vi "4_Meas_Tdon.vi"(5 "Request #":string, 6 "TEST #":string, 7 "Project #":string, 8 "error in (no error)":errorcluster, 9 "ICE":dbl, 10 "VGE":dbl, 11 "file path (IN)":path) -> (0 "error out":errorcluster, 1 "DONE Tdon":bool, 2 "Tdon (ns)":dbl, 3 "file path (OUT)":path, 4 "ON Region":waveform(dbl)[](graph) caption="Tdon (ns)")   [LabVIEW 2020]
uses:
  <vilib>/Waveform/WDTOps.llb/WDT Waveform Duration DBL.vi
  <vilib>/Waveform/WDTOps.llb/WDT Get Waveform Subset DBL.vi
  <vilib>/measure/mascope.llb/Transition Measurements 1 chan.vi
  <vilib>/measure/NI_MAPro.lvlib
panel:
  out "Cursor a : Channel 2":dbl
  out "Cursor a : Channel 1":dbl
  in  "Decision ?":bool
  in  "Cursor a : Channel 1 \nrise edge tolerance":dbl=0.1
  in  "Cursor a : Channel 1 \nrise edge number":i32=1
  in  "Cursor a : Channel 2\nrise edge tolerance":dbl=0.1
  in  "Cursor a : Channel 2\nrise edge number":i32=1
  in  "reference  levels (CH1 initialize)":T1={"high ref level"=90.0, "mid ref level"=50.0, "low ref level"=10.0, "ref units"=1} {"ref units" items=["absolute", "percent"]; "high ref level" format="%0.2f"; "low ref level" format="%0.2f"; "mid ref level" format="%0.2f"}
  in  "reference  levels (CH2 initialize)":T1={"high ref level"=90.0, "mid ref level"=50.0, "low ref level"=10.0, "ref units"=1} {"ref units" items=["absolute", "percent"]; "high ref level" format="%0.2f"; "low ref level" format="%0.2f"; "mid ref level" format="%0.2f"}
  out "measurement info (CH2)":T2 {"ref levels"."ref units" items=["absolute", "relative"]; "ref levels"."high ref level" format="%.2p"; "ref levels"."low ref level" format="%.2p"; "ref levels"."mid ref level" format="%.2p"; "end time" format="%.6e"; "start time" format="%.6e"}
  out "measurement info (CH1)":T2 {"ref levels"."ref units" items=["absolute", "relative"]; "ref levels"."high ref level" format="%.2p"; "ref levels"."low ref level" format="%.2p"; "ref levels"."mid ref level" format="%.2p"; "end time" format="%.6e"; "start time" format="%.6e"}
  out "10% Vge":dbl
  out "10% Ice":dbl
  out "Waveform Graph":waveform(dbl)[](graph)
  # "From 10% Vge to 10% Ice"
  # "\"ON Region\" Test"
  # "From 10% Vge to 10% Ice"
  # "Default = 1"
  # "Default = 1"
  # "Default = 0.1"
  # "Default = 0.1"
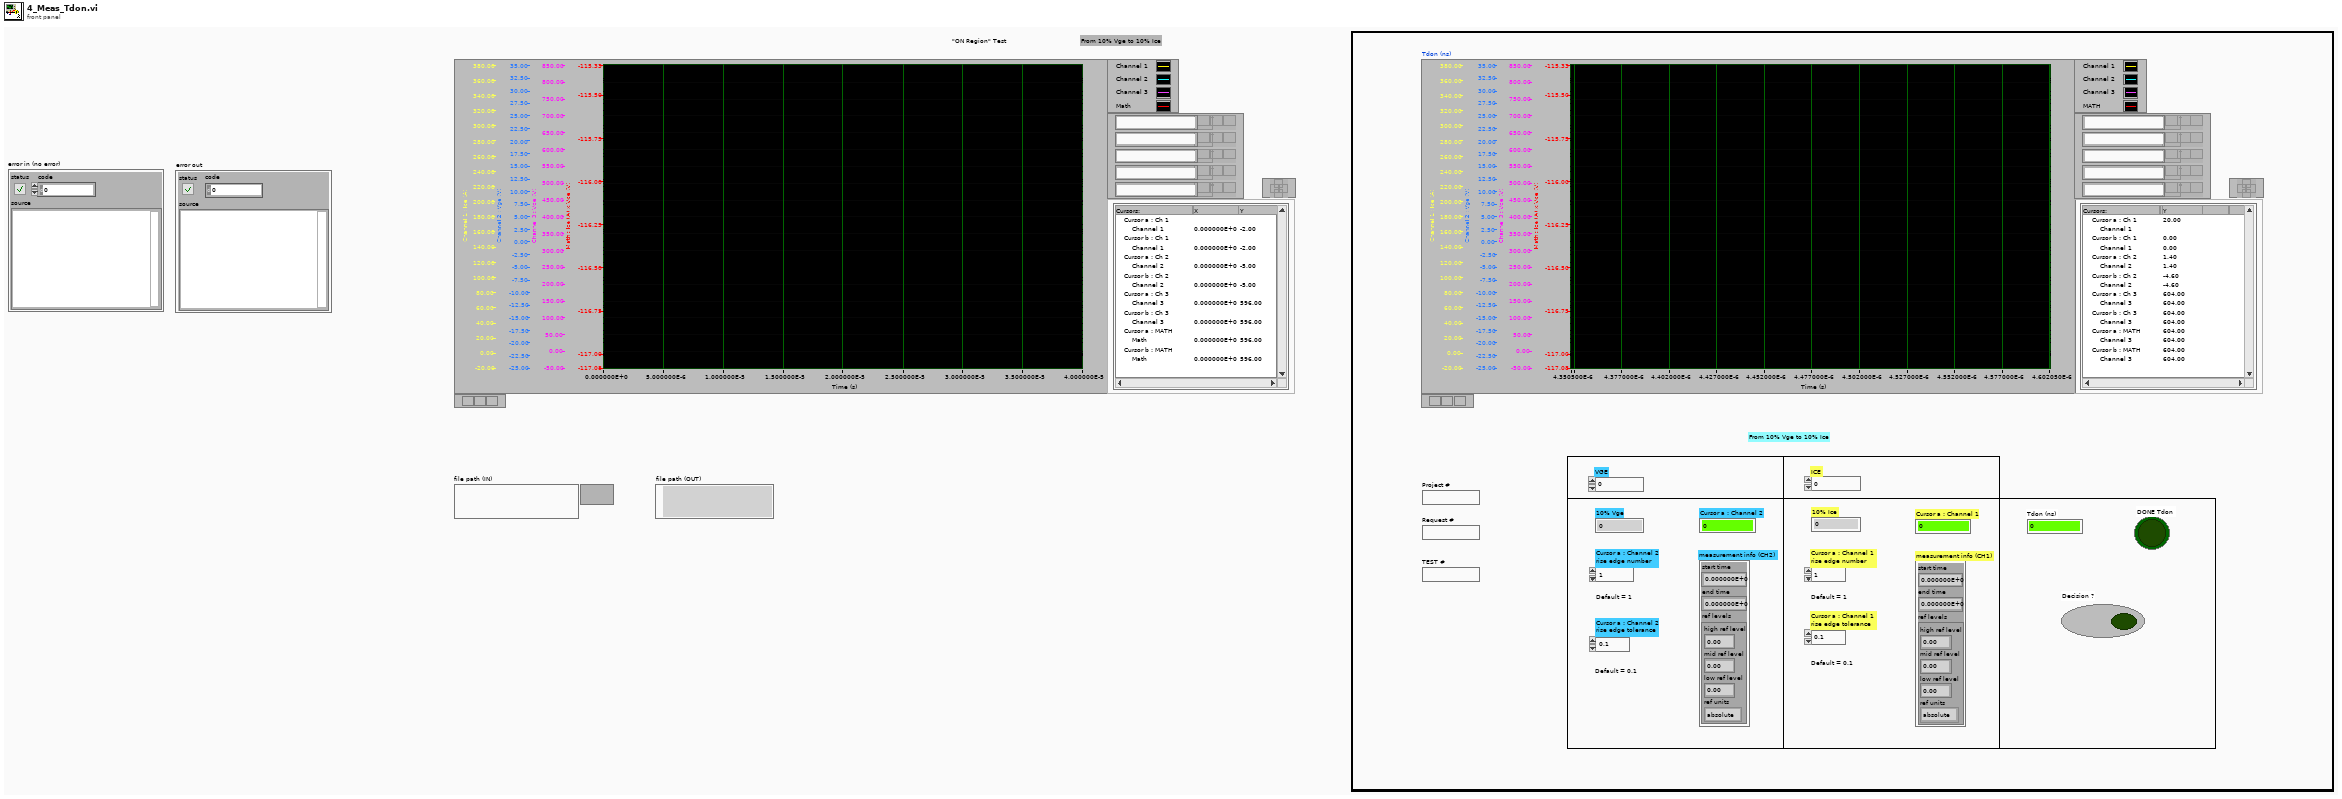
[diagram p1: front panel]
types:
  T1 = cluster{"high ref level":dbl, "mid ref level":dbl, "low ref level":dbl, "ref units":u16}
  T2 = cluster{"start time":dbl, "end time":dbl, "ref levels":cluster{"high ref level":dbl, "mid ref level":dbl, "low ref level":dbl, "ref units":u16}}
  T3 = enum32{"Invalid", "Standard", "Closed", "Hidden", "Minimized", "Maximized"}
  T4 = typedef "imagedata.ctl" = cluster{"image type":i32, "image depth":i32, "image":u8[], "mask":u8[], "colors":u32[], "Rectangle":cluster{"left":i16, "top":i16, "right":i16, "bottom":i16}}
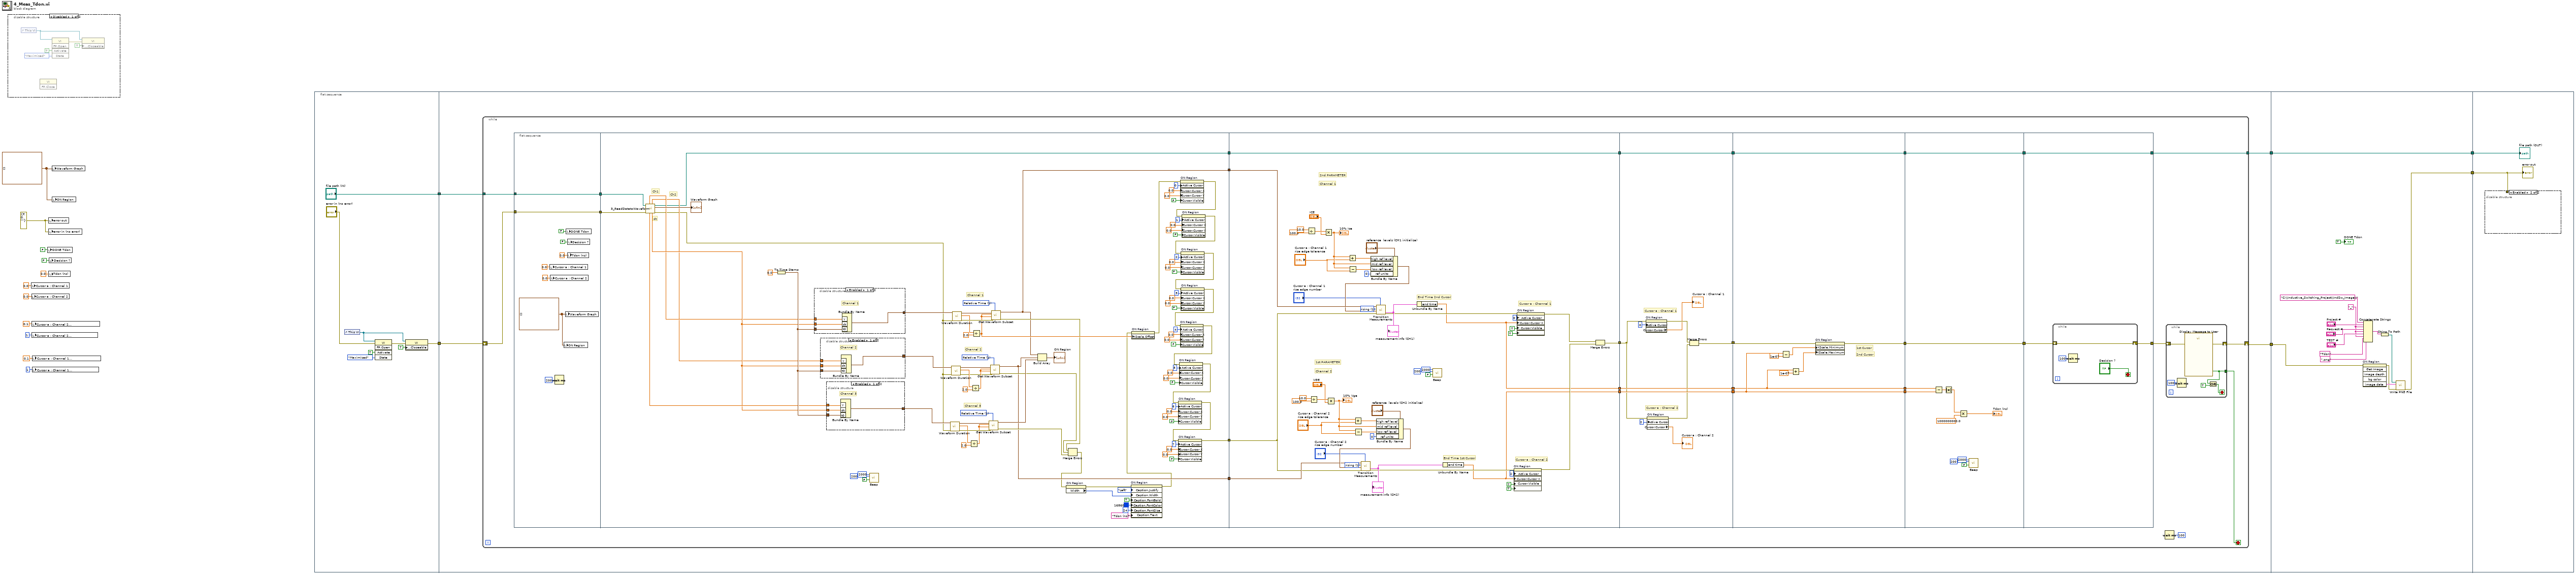
[diagram p0: block diagram]
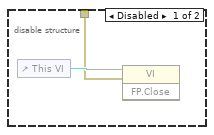
[diagram p6: hidden frame]
diagram:
  w16 = errorcluster {"status"=FALSE, "code"=0, "source"=""} ("error out")
  w17 = waveform(dbl)[] [] ("Waveform Graph")
  n1 = disable-structure shown="Disabled" {
    frame Disabled {
      n2 = control-ref of="This VI"() -> (w19:refnum<vi>)
      n3 = invoke class="VI" method="FP.Close"() -> (reference=w18:refnum<vi>)  [unwired: 2 in, 3 out]
      n4 = invoke class="VI" method="FP.Open"(reference=w19, "Activate"=TRUE ("Activate?"), "State"=T3."Maximized") -> (error in=w22:errorcluster, error out=w20:errorcluster)  [unwired: 1 in, 4 out]
      n5 = property class="VI"(reference=w19, error in=w20, "Front Panel.Closeable"=TRUE ("Front Panel Window:Closeable")) -> ()  [unwired: 2 out]
    }
    frame Enabled {
    }
  }
  n6 = local write "Cursor a : Channel 1"(0.0 ("Cursor a : Channel 1")) -> ()
  n7 = local write "Cursor a : Channel 2"(0.0 ("Cursor a : Channel 2")) -> ()
  n8 = local write "Cursor a : Channel 2\nrise edge tolerance"(0.1 ("Cursor a : Channel 2\nrise edge tolerance")) -> ()
  n9 = local write "Cursor a : Channel 2\nrise edge number"(1 ("Cursor a : Channel 2\nrise edge number")) -> ()
  n10 = local write "Cursor a : Channel 1 \nrise edge tolerance"(0.1 ("Cursor a : Channel 1 \nrise edge tolerance")) -> ()
  n11 = local write "Cursor a : Channel 1 \nrise edge number"(1 ("Cursor a : Channel 1 \nrise edge number")) -> ()
  n12 = local write "DONE Tdon"(FALSE ("DONE Tdon")) -> ()
  n13 = local write "error out"(w16) -> ()
  n14 = local write "error in (no error)"(w16) -> ()
  n15 = local write "Tdon (ns)"(0.0 ("Tdon (ns)")) -> ()
  n16 = local write "Decision ?"(FALSE ("Decision ?")) -> ()
  n17 = local write "Waveform Graph"(w17) -> ()
  n18 = local write "ON Region"(w17) -> ()
  n19 = flat-sequence {
    tunnel: ["file path (IN)"] -> w6
    tunnel: [w27] -> w5
    tunnel: [w35] -> w15
    tunnel: [w34] -> w12
    tunnel: w6 -> [w36]
    tunnel: w5 -> [w33]
    tunnel: w15 -> [w270]
    tunnel: [w269] -> w14
    tunnel: [w268] -> w13
    tunnel: w12 -> [w268]
    tunnel: w14 -> [w283]
    tunnel: w13 -> [w284]
    frame #0 {
      n20 = control-ref of="This VI"() -> (w31:refnum<vi>)
      n21 = invoke class="VI" method="FP.Open"(reference=w31, error in="error in (no error)", "Activate"=TRUE ("Activate?"), "State"=T3."Maximized") -> (error out=w32:errorcluster)  [unwired: 1 in, 4 out]
      n22 = property class="VI"(reference=w31, error in=w32, "Front Panel.Closeable"=TRUE ("Front Panel Window:Closeable")) -> (error out=w27:errorcluster)  [unwired: 1 out]
    }
    frame #1 {
      n23 = while {
        tunnel: w36 -> [w52]
        shift-right: [w38] -> w35
        shift-left: w33 -> [w50]
        tunnel: [w48] -> w34
        stop <- w37 stop-if-true
        n24 = flat-sequence {
          tunnel: [w77] -> w63
          tunnel: [w78] -> w62
          tunnel: w52 -> [w78]
          tunnel: w50 -> [w77]
          tunnel: w63 -> [w170]
          tunnel: w62 -> [w164]
          tunnel: [w91] -> w61
          tunnel: [w90] -> w60
          tunnel: [w89] -> w59
          tunnel: [w79] -> w58
          tunnel: w61 -> [w207]
          tunnel: w60 -> [w206]
          tunnel: w59 -> [w205]
          tunnel: [w193] -> w47
          tunnel: [w192] -> w45
          tunnel: [w191] -> w43
          tunnel: w58 -> [w190]
          tunnel: [w190] -> w41
          tunnel: w47 -> [w241]
          tunnel: [w241] -> w46
          tunnel: w45 -> [w240]
          tunnel: [w240] -> w44
          tunnel: w43 -> [w235]
          tunnel: [w238] -> w42
          tunnel: w41 -> [w239]
          tunnel: [w239] -> w40
          tunnel: w46 -> [w242]
          tunnel: [w242] -> w57
          tunnel: w44 -> [w243]
          tunnel: [w243] -> w56
          tunnel: w42 -> [w249]
          tunnel: [w248] -> w55
          tunnel: w40 -> [w250]
          tunnel: [w250] -> w54
          tunnel: w57 -> [w260]
          tunnel: w56 -> [w259]
          tunnel: w55 -> [w252]
          tunnel: w54 -> [w251]
          tunnel: [w252] -> w53
          tunnel: [w251] -> w49
          tunnel: w53 -> [w264]
          tunnel: [w263] -> w39
          tunnel: w49 -> [w262]
          tunnel: [w262] -> w48
          frame #0 {
            w73 = waveform(dbl)[] [] ("Waveform Graph")
            n25 = local write "Cursor a : Channel 1"(0.0 ("Cursor a : Channel 1")) -> ()
            n26 = local write "Cursor a : Channel 2"(0.0 ("Cursor a : Channel 2")) -> ()
            n27 = Wait (ms)(milliseconds to wait=u32 200) -> ()  [unwired: 1 out]
            n28 = local write "ON Region"(w73) -> ()
            n29 = local write "Waveform Graph"(w73) -> ()
            n30 = local write "DONE Tdon"(FALSE ("DONE Tdon")) -> ()
            n31 = local write "Tdon (ns)"(0.0 ("Tdon (ns)")) -> ()
            n32 = local write "Decision ?"(FALSE ("Decision ?")) -> ()
          }
          frame #1 {
            w145 = u16 1 items=["Samples", "Relative Time"] ("start/duration format")
            w156 = u16 1 items=["Samples", "Relative Time"] ("start/duration format")
            w157 = u16 1 items=["Samples", "Relative Time"] ("start/duration format")
            # "Channel 1"
            # "Channel 3"
            # "Channel 2"
            # "dt"
            # "Ch2"
            # "Ch1"
            n33 = call "3_ReadDatatoWaveform.vi"("error in (no error)"=w170, "file path (IN)"=w164) -> ("error out"=w138:errorcluster, "Waveform Graph"=→"Waveform Graph":waveform(dbl)[], "file path (OUT)"=w79:path, "dt"=w165:dbl, "Ch 2 Data"=w162:dbl[], "Ch 3 Data"=w166:dbl[], "Ch 1 Data"=w163:dbl[])  [unwired: 3 in]
            n34 = To Time Stamp(1:0.0 ("number")) -> (0:w167:timestamp)
            n35 = disable-structure shown="Enabled" {
              disable-tunnel: w167 -> [w174 _]
              disable-tunnel: w165 -> [w173 _]
              disable-tunnel: w163 -> [w172 _]
              disable-tunnel: [w171 _] -> w144
              frame Enabled {
                # "Channel 1"
                n36 = Bundle By Name("Y"=w172, "dt"=w173, "t0"=w174) -> (w171:waveform(dbl))  [unwired: 1 in]
              }
              frame Disabled {
              }
            }
            n37 = disable-structure shown="Enabled" {
              disable-tunnel: w167 -> [w178 _]
              disable-tunnel: w165 -> [w177 _]
              disable-tunnel: w162 -> [w176 _]
              disable-tunnel: [w175 _] -> w143
              frame Enabled {
                # "Channel 2"
                n38 = Bundle By Name("Y"=w176, "dt"=w177, "t0"=w178) -> (w175:waveform(dbl))  [unwired: 1 in]
              }
              frame Disabled {
              }
            }
            n39 = disable-structure shown="Enabled" {
              disable-tunnel: w167 -> [w182 _]
              disable-tunnel: w165 -> [w181 _]
              disable-tunnel: w166 -> [w180 _]
              disable-tunnel: [w179 _] -> w142
              frame Enabled {
                # "Channel 3"
                n40 = Bundle By Name("Y"=w180, "dt"=w181, "t0"=w182) -> (w179:waveform(dbl))  [unwired: 1 in]
              }
              frame Disabled {
              }
            }
            n41 = call <vilib>:"Beep.vi"("use system alert? (T)"=FALSE, "duration (msec)"=u32 200, "frequency (Hz)"=u32 2000) -> ()  [unwired: 9 in]
            n42 = call-poly <vilib>:"Waveform Duration.vi"("error in (no error)"=w138, "waveform in"=w142) -> ("error out"=w150:errorcluster, "duration"=w147:dbl, "waveform out"=w149:waveform(dbl))  [unwired: 7 in]
            n43 = call-poly <vilib>:"Waveform Duration.vi"("error in (no error)"=w138, "waveform in"=w143) -> ("error out"=w151:errorcluster, "duration"=w154:dbl, "waveform out"=w152:waveform(dbl))  [unwired: 7 in]
            n44 = call-poly <vilib>:"Waveform Duration.vi"("error in (no error)"=w138, "waveform in"=w144) -> ("error out"=w161:errorcluster, "duration"=w158:dbl, "waveform out"=w160:waveform(dbl))  [unwired: 7 in]
            n45 = Divide(x=w147, y=2.0) -> (x/y=w146:dbl)
            n46 = Divide(x=w154, y=2.0) -> (x/y=w155:dbl)
            n47 = Divide(x=w158, y=2.0) -> (x/y=w139:dbl)
            n48 = call-poly <vilib>:"Get Waveform Subset.vi"("start/duration format"=w145, "error in (no error)"=w150, "duration"=w146, "start samples/time"=w146, "waveform in"=w149) -> ("error out"=w135:errorcluster, "waveform out"=w141:waveform(dbl))  [unwired: 1 in, 2 out]
            n49 = call-poly <vilib>:"Get Waveform Subset.vi"("start/duration format"=w156, "error in (no error)"=w151, "duration"=w155, "start samples/time"=w155, "waveform in"=w152) -> ("error out"=w136:errorcluster, "waveform out"=w91:waveform(dbl))  [unwired: 1 in, 2 out]
            n50 = call-poly <vilib>:"Get Waveform Subset.vi"("start/duration format"=w157, "error in (no error)"=w161, "duration"=w139, "start samples/time"=w139, "waveform in"=w160) -> ("error out"=w137:errorcluster, "waveform out"=w90:waveform(dbl))  [unwired: 1 in, 2 out]
            n51 = Build Array(w90, w91, w141) -> (→"ON Region":waveform(dbl)[])
            n52 = Merge Errors(w137, w136, w135) -> (w87:errorcluster)
            n53 = property on="ON Region" class="WFGraph (strict)"(error in=w87) -> (error out=w86:errorcluster, "Width"=w85:u32)  [unwired: 1 in, 1 out]
            n54 = property on="ON Region" class="WFGraph (strict)"(error in=w86, "Caption.Justify"=enum16{"Left", "Center", "Right"}."Left" ("Caption.Justification"), "Caption.Width"=w85, "Caption.FontBold"=TRUE ("Caption.Font:Bold"), "Caption.FontColor"=u32 16860 ("Caption.Font:Color"), "Caption.FontSize"=u32 24 ("Caption.Font:Size"), "Caption.Text"="Tdon (ns)") -> (error out=w81:errorcluster)  [unwired: 1 in, 1 out]
            n55 = property on="ON Region" class="WFGraph (strict)"(error in=w81, "XScale.Offset"=w139) -> (error out=w115:errorcluster)  [unwired: 1 in, 1 out]
            n56 = property on="ON Region" class="WFGraph (strict)"(error in=w115, "Active Cursor"=u32 0, "Cursor.Cursor X"=0.0 ("Cursor.Cursor Position:Cursor X"), "Cursor.Cursor Y"=0.0 ("Cursor.Cursor Position:Cursor Y"), "Cursor.Visible"=FALSE) -> (error out=w114:errorcluster)  [unwired: 1 in, 1 out]
            n57 = property on="ON Region" class="WFGraph (strict)"(error in=w114, "Active Cursor"=u32 1, "Cursor.Cursor X"=0.0 ("Cursor.Cursor Position:Cursor X"), "Cursor.Cursor Y"=0.0 ("Cursor.Cursor Position:Cursor Y"), "Cursor.Visible"=FALSE) -> (error out=w113:errorcluster)  [unwired: 1 in, 1 out]
            n58 = property on="ON Region" class="WFGraph (strict)"(error in=w113, "Active Cursor"=u32 2, "Cursor.Cursor X"=0.0 ("Cursor.Cursor Position:Cursor X"), "Cursor.Cursor Y"=0.0 ("Cursor.Cursor Position:Cursor Y"), "Cursor.Visible"=FALSE) -> (error out=w112:errorcluster)  [unwired: 1 in, 1 out]
            n59 = property on="ON Region" class="WFGraph (strict)"(error in=w112, "Active Cursor"=u32 3, "Cursor.Cursor X"=0.0 ("Cursor.Cursor Position:Cursor X"), "Cursor.Cursor Y"=0.0 ("Cursor.Cursor Position:Cursor Y"), "Cursor.Visible"=FALSE) -> (error out=w95:errorcluster)  [unwired: 1 in, 1 out]
            n60 = property on="ON Region" class="WFGraph (strict)"(error in=w95, "Active Cursor"=u32 4, "Cursor.Cursor X"=0.0 ("Cursor.Cursor Position:Cursor X"), "Cursor.Cursor Y"=0.0 ("Cursor.Cursor Position:Cursor Y"), "Cursor.Visible"=FALSE) -> (error out=w94:errorcluster)  [unwired: 1 in, 1 out]
            n61 = property on="ON Region" class="WFGraph (strict)"(error in=w94, "Active Cursor"=u32 5, "Cursor.Cursor X"=0.0 ("Cursor.Cursor Position:Cursor X"), "Cursor.Cursor Y"=0.0 ("Cursor.Cursor Position:Cursor Y"), "Cursor.Visible"=FALSE) -> (error out=w93:errorcluster)  [unwired: 1 in, 1 out]
            n62 = property on="ON Region" class="WFGraph (strict)"(error in=w93, "Active Cursor"=u32 6, "Cursor.Cursor X"=0.0 ("Cursor.Cursor Position:Cursor X"), "Cursor.Cursor Y"=0.0 ("Cursor.Cursor Position:Cursor Y"), "Cursor.Visible"=FALSE) -> (error out=w92:errorcluster)  [unwired: 1 in, 1 out]
            n63 = property on="ON Region" class="WFGraph (strict)"(error in=w92, "Active Cursor"=u32 7, "Cursor.Cursor X"=0.0 ("Cursor.Cursor Position:Cursor X"), "Cursor.Cursor Y"=0.0 ("Cursor.Cursor Position:Cursor Y"), "Cursor.Visible"=FALSE) -> (error out=w89:errorcluster)  [unwired: 1 in, 1 out]
          }
          frame #2 {
            w221 = u16 1 items=["falling", "rising"] ("polarity (rising)")
            w222 = u16 1 items=["falling", "rising"] ("polarity (rising)")
            # "Cursor a : Channel 2"
            # "Cursor a : Channel 1"
            # "End Time 2nd Cursor"
            # "End Time 1st Cursor"
            # "2nd PARAMETER"
            # "Channel 1"
            # "1st PARAMETER"
            # "Channel 2"
            n64 = Divide(x=10.0, y=100.0) -> (x/y=w230:dbl)
            n65 = Divide(x=10.0, y=100.0) -> (x/y=w226:dbl)
            n66 = Multiply(x=w230, y="ICE") -> (x*y=w208:dbl)
            "10% Ice" <- w208
            n67 = Multiply(x=w226, y="VGE") -> (x*y=w214:dbl)
            "10% Vge" <- w214
            n68 = Add(x=w208, y="Cursor a : Channel 1 \nrise edge tolerance") -> (x+y=w213:dbl)
            n69 = Subtract(x=w208, y="Cursor a : Channel 1 \nrise edge tolerance") -> (x-y=w212:dbl)
            n70 = Add(x=w214, y="Cursor a : Channel 2\nrise edge tolerance") -> (x+y=w220:dbl)
            n71 = Subtract(x=w214, y="Cursor a : Channel 2\nrise edge tolerance") -> (x-y=w219:dbl)
            n72 = Bundle By Name(cluster="reference  levels (CH1 initialize)", "high ref level"=w213, "mid ref level"=w208, "low ref level"=w212, "ref units"=u16 0) -> (w185:T1)
            n73 = call-poly <vilib>:"Transition Measurements.vi"("edge number (1)"="Cursor a : Channel 1 \nrise edge number", "error in (no error)"=w205, "reference levels"=w185, "polarity (rising)"=w222, "signal in"=w206) -> ("error out"=w202:errorcluster, "measurement info"=w209:T2)  [unwired: 1 in, 4 out]
            "measurement info (CH1)" <- w209
            n74 = Bundle By Name(cluster="reference  levels (CH2 initialize)", "high ref level"=w220, "mid ref level"=w214, "low ref level"=w219, "ref units"=u16 0) -> (w216:T1)
            n75 = call-poly <vilib>:"Transition Measurements.vi"("edge number (1)"="Cursor a : Channel 2\nrise edge number", "error in (no error)"=w205, "reference levels"=w216, "polarity (rising)"=w221, "signal in"=w207) -> ("error out"=w199:errorcluster, "measurement info"=w215:T2)  [unwired: 1 in, 4 out]
            "measurement info (CH2)" <- w215
            n76 = Unbundle By Name(w209) -> ("end time"=w193:dbl)
            n77 = call <vilib>:"Beep.vi"("use system alert? (T)"=FALSE, "duration (msec)"=u32 200, "frequency (Hz)"=u32 2000) -> ()  [unwired: 9 in]
            n78 = Unbundle By Name(w215) -> ("end time"=w192:dbl)
            n79 = property on="ON Region" class="WFGraph (strict)"(error in=w199, "Active Cursor"=u32 2, "Cursor.Cursor X"=w192, "Cursor.Visible"=TRUE, "Cursor.Cursor Name Visible"=TRUE) -> (error out=w194:errorcluster)  [unwired: 1 in, 1 out]
            n80 = property on="ON Region" class="WFGraph (strict)"(error in=w202, "Active Cursor"=u32 0, "Cursor.Cursor X"=w193, "Cursor.Visible"=TRUE, "Cursor.Cursor Name Visible"=TRUE) -> (error out=w195:errorcluster)  [unwired: 1 in, 1 out]
            n81 = Merge Errors(w195, w194) -> (w191:errorcluster)
          }
          frame #3 {
            # "Cursor a : Channel 2"
            # "Cursor a : Channel 1"
            n82 = property on="ON Region" class="WFGraph (strict)"(error in=w235, "Active Cursor"=u32 0) -> (error out=w234:errorcluster, "Cursor.Cursor Y"=→"Cursor a : Channel 1":dbl)  [unwired: 1 in, 1 out]
            n83 = property on="ON Region" class="WFGraph (strict)"(error in=w235, "Active Cursor"=u32 2) -> (error out=w233:errorcluster, "Cursor.Cursor Y"=→"Cursor a : Channel 2":dbl)  [unwired: 1 in, 1 out]
            n84 = Merge Errors(w234, w233) -> (w238:errorcluster)
          }
          frame #4 {
            # "2nd Cursor"
            # "1st Cursor"
            n85 = Subtract(x=w243, y=1e-07) -> (x-y=w246:dbl)
            n86 = Add(x=w242, y=1e-07) -> (x+y=w244:dbl)
            n87 = property on="ON Region" class="WFGraph (strict)"(error in=w249, "XScale.Minimum"=w246, "XScale.Maximum"=w244) -> (error out=w248:errorcluster)  [unwired: 1 in, 1 out]
          }
          frame #5 {
            n88 = Subtract(x=w260, y=w259) -> (x-y=w254:dbl)
            n89 = Absolute Value(x=w254) -> (abs(x)=w253:dbl)
            n90 = Multiply(x=w253, y=1000000000.0) -> (x*y=→"Tdon (ns)":dbl)
            n91 = call <vilib>:"Beep.vi"("use system alert? (T)"=FALSE, "duration (msec)"=u32 200, "frequency (Hz)"=u32 2000) -> ()  [unwired: 9 in]
          }
          frame #6 {
            n92 = while {
              shift-right: [w265] -> w263
              shift-left: w264 -> [w265]
              stop <- "Decision ?" stop-if-true
              n93 = Wait (ms)(milliseconds to wait=u32 100) -> ()  [unwired: 1 out]
            }
          }
        }
        n94 = Wait (ms)(milliseconds to wait=u32 100) -> ()  [unwired: 1 out]
        n95 = while {
          tunnel: [w65] -> w37
          shift-right: [w68] -> w38
          shift-left: w39 -> [w69]
          stop <- w67 stop-if-true
          n96 = Wait (ms)(milliseconds to wait=u32 100) -> ()  [unwired: 1 out]
          n97 = call "Display Message to User"("error in (no error)"=w69) -> ("error out"=w68:errorcluster, "NO"=w65:bool)  [unwired: 9 in]
          n98 = Or(x=w65, y=TRUE) -> (x .or. y?=w67:bool)
        }
      }
    }
    frame #2 {
      w273 = "_"
      n99 = invoke on="ON Region" class="WFGraph (strict)" method="Get Image"(error in=w270) -> (error out=w276:errorcluster, "image data"=w279:T4)  [unwired: 5 in, 4 out]
      n100 = Concatenate Strings("C:\\Inductive_Switching_Project\\IndSw_Image\\" ("string"), "Project #", w273, "Request #", w273, "TEST #", w273, "Tdon" ("string"), ".png" ("string")) -> (w280:string)
      n101 = String To Path(string=w280) -> (path=w278:path)
      n102 = call <vilib>:"Write PNG File.vi"("error in (no error)"=w276, "image data"=w279, "path to PNG file"=w278) -> ("error out"=w269:errorcluster)  [unwired: 7 in, 1 out]
      "DONE Tdon" <- TRUE ("DONE Tdon")
    }
    frame #3 {
      n103 = disable-structure shown="Enabled" {
        disable-tunnel: w283 -> [w285 _]
        frame Disabled {
          n104 = control-ref of="This VI"() -> (w286:refnum<vi>)
          n105 = invoke class="VI" method="FP.Close"(reference=w286, error in=w285) -> ()  [unwired: 1 in, 3 out]
        }
        frame Enabled {
        }
      }
      "error out" <- w283
      "file path (OUT)" <- w284
    }
  }
